vi "Sub Build Json String.vi"(8 "error in (no error)":errorcluster, 11 "Pic Json Generator in":refnum<class "Pic Json Generator.lvclass">) -> (0 "error out":errorcluster, 2 "Json String":string, 3 "Pic Json Generator out":refnum<class "Pic Json Generator.lvclass">)   [LabVIEW 2018, in "Pic Json Generator.lvlib" / "Pic Json Generator.lvclass"]
uses:
  Pic Json Generator.lvclass
  Pic Json Generator.lvclass/Pic Json Generator.ctl
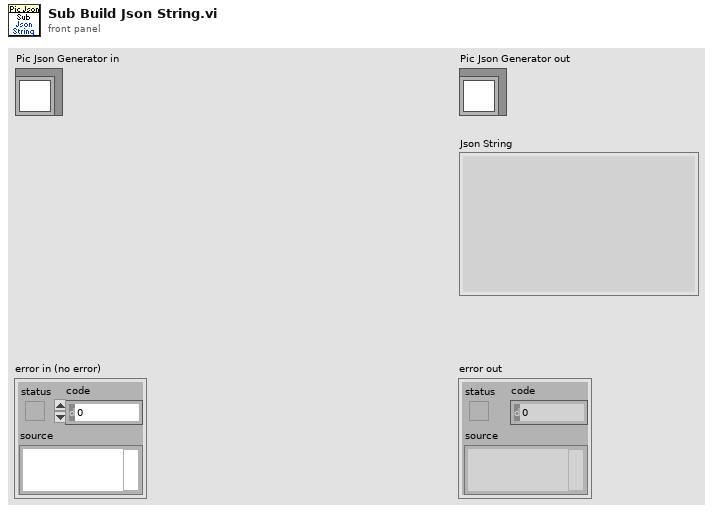
[diagram p1: front panel]
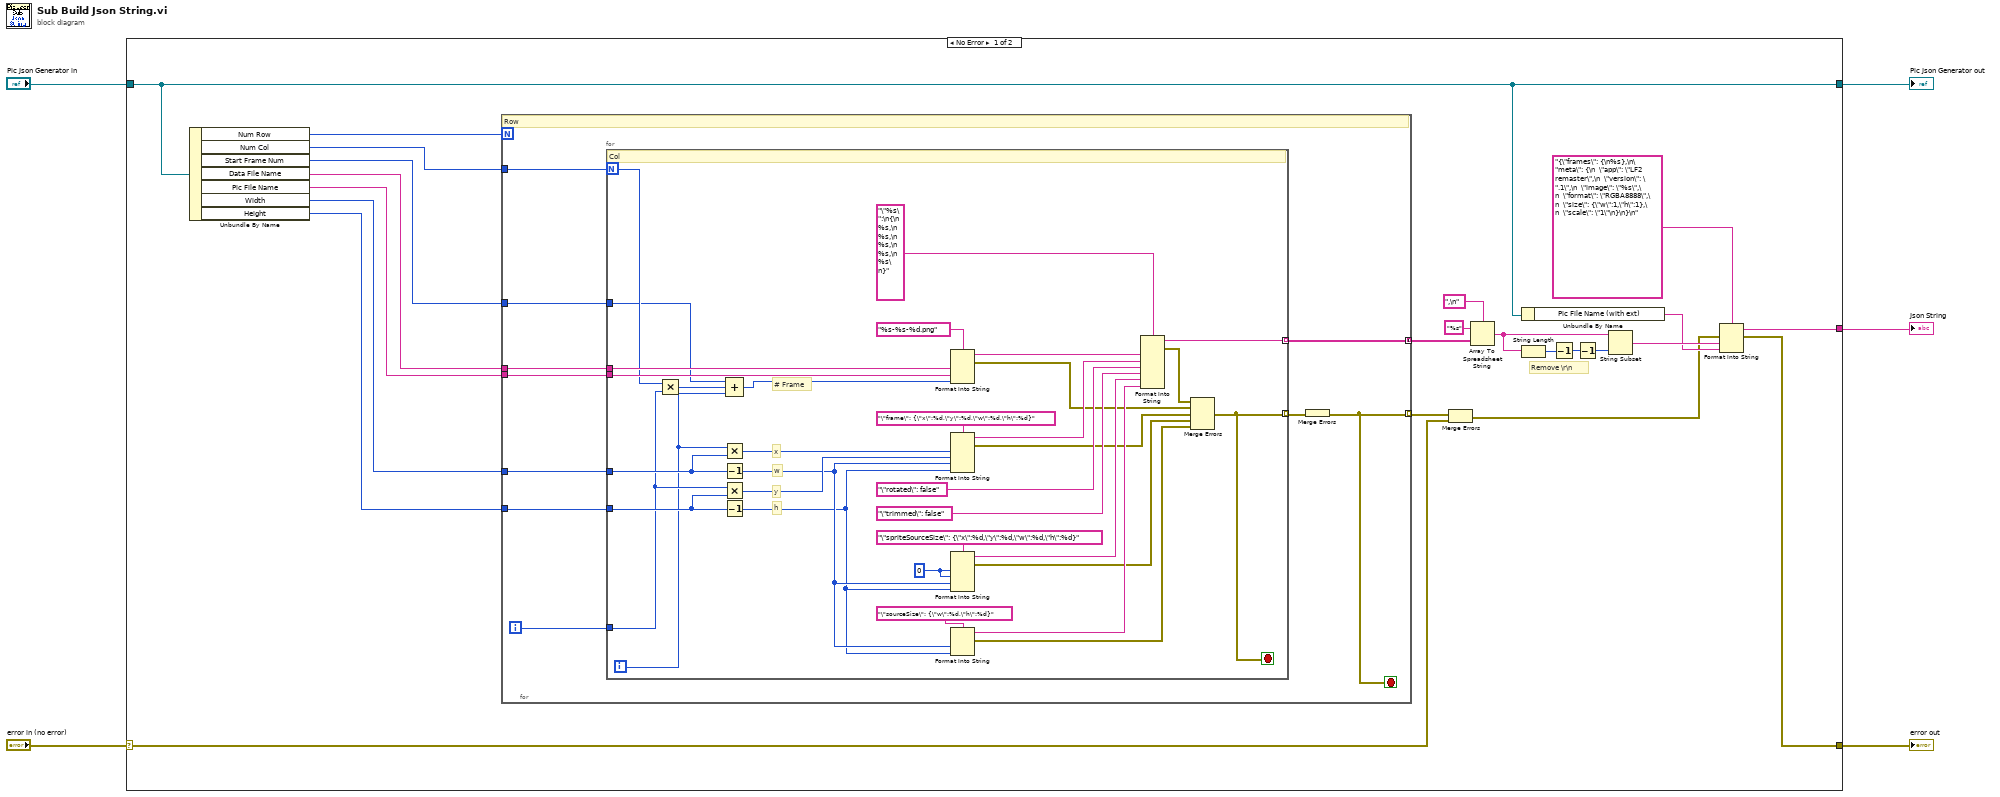
[diagram p0: block diagram]
diagram:
  n1 = case shown="No Error" "error in (no error)" {
    selector: "error in (no error)" -> [w20 w73]
    tunnel: [w7 w73] -> w2
    tunnel: [w10 w72] -> w3
    tunnel: "Pic Json Generator in" -> [w10 w72]
    tunnel: [w6 _] -> w1
    frame No Error {
      # "Remove \\r\\n"
      n2 = Unbundle By Name(w10) -> ("Num Row"=w28:u32, "Num Col"=w27:u32, "Start Frame Num"=w26:u32, "Data File Name"=w25:string, "Pic File Name"=w24:string, "Width"=w23:u32, "Height"=w22:u32)
      n3 = for {
        N: w28 -> [_]
        tunnel: w25 -> [w38]
        tunnel: w24 -> [w37]
        tunnel: w23 -> [w34]
        tunnel: w22 -> [w33]
        tunnel: w27 -> [w36]
        tunnel: [w32] -> w13 mode=concatenating
        tunnel: w26 -> [w31]
        tunnel: [w29] -> w21 mode=indexing
        i -> [w35]
        stop <- w29 stop-if-true
        # "Row"
        n4 = for {
          N: w36 -> [w46]
          tunnel: w38 -> [w71]
          tunnel: w37 -> [w70]
          tunnel: w35 -> [w63]
          tunnel: w34 -> [w66]
          tunnel: w33 -> [w64]
          tunnel: [w50] -> w32 mode=indexing
          tunnel: w31 -> [w45]
          tunnel: [w39] -> w30 mode=indexing
          i -> [w49]
          stop <- w39 stop-if-true
          w61 = 0 ("input 1")
          # "# Frame"
          # "h"
          # "w"
          # "y"
          # "x"
          # "Col"
          n5 = Multiply(x=w46, y=w63) -> (x*y=w48:i32)
          n6 = Multiply(x=w49, y=w66) -> (x*y=w65:u32)
          n7 = Decrement(x=w66) -> (x-1=w59:u32)
          n8 = Multiply(x=w63, y=w64) -> (x*y=w62:u32)
          n9 = Decrement(x=w64) -> (x-1=w58:u32)
          n10 = Compound Arithmetic op=ADD(w45, w48, w49) -> (w47:u32)
          n11 = Format Into String(format string="%s-%s-%d.png", w71, w70, w47) -> (resulting string=w56:string, error out=w43:errorcluster)  [unwired: 2 in]
          n12 = Format Into String(format string="\"frame\": {\"x\":%d,\"y\":%d,\"w\":%d,\"h\":%d}", w65, w62, w59, w58) -> (resulting string=w55:string, error out=w42:errorcluster)  [unwired: 2 in]
          n13 = Format Into String(format string="\"spriteSourceSize\": {\"x\":%d,\"y\":%d,\"w\":%d,\"h\":%d}", w61, w61, w59, w58) -> (resulting string=w52:string, error out=w41:errorcluster)  [unwired: 2 in]
          n14 = Format Into String(format string="\"sourceSize\": {\"w\":%d,\"h\":%d}", w59, w58) -> (resulting string=w51:string, error out=w40:errorcluster)  [unwired: 2 in]
          n15 = Format Into String(format string="\"%s\":\n{\n  %s,\n  %s,\n  %s,\n  %s,\n  %s\n}", w56, w55, "\"rotated\": false" ("format string"), "\"trimmed\": false" ("format string"), w52, w51) -> (resulting string=w50:string, error out=w44:errorcluster)  [unwired: 2 in]
          n16 = Merge Errors(w44, w43, w42, w41, w40) -> (w39:errorcluster)
        }
        n17 = Merge Errors(w30) -> (w29:errorcluster)
      }
      n18 = Merge Errors(w21, w20) -> (w8:errorcluster)
      n19 = Array To Spreadsheet String(delimiter (Tab)=",\n", array=w13, 3:"%s" ("format string")) -> (spreadsheet string=w16:string)
      n20 = Unbundle By Name(w10) -> ("Pic File Name (with ext)"=w9:string)
      n21 = String Length(string=w16) -> (length=w17:i32)
      n22 = Decrement(x=w17) -> (x-1=w15:i32)
      n23 = Decrement(x=w15) -> (x-1=w14:i32)
      n24 = String Subset(string=w16, length (rest)=w14) -> (substring=w11:string)  [unwired: 1 in]
      n25 = Format Into String(format string="{\"frames\": {\n%s},\n\"meta\": {\n  \"app\": \"LF2 remaster\",\n  \"version\": \".1\",\n  \"image\": \"%s\",\n  \"format\": \"RGBA8888\",\n  \"size\": {\"w\":1,\"h\":1},\n  \"scale\": \"1\"\n}\n}\n", error in=w8, w11, w9) -> (resulting string=w6:string, error out=w7:errorcluster)  [unwired: 1 in]
    }
    frame Error {
    }
  }
  "error out" <- w2
  "Pic Json Generator out" <- w3
  "Json String" <- w1
